vi "LIN To 2SCU.vi"() -> ()   [LabVIEW 2018]
panel:
  in  "NAD":u8[](array[numeric])=[13, 120] format="%.0x"
  in  "关闭卷帘":bool
  in  "展开卷帘":bool
  in  "关闭天窗":bool
  in  "打开天窗":bool
  in  "Send":bool
  out "Tx Rx Data":string
  out "Response Good?":bool
  in  "Exit":bool
  in  "interface":refnum<k21>="LIN2"
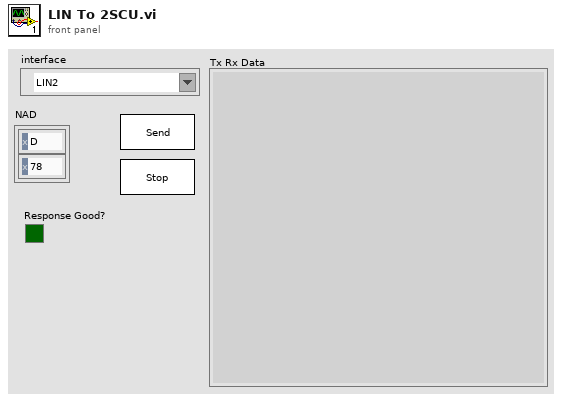
[diagram p1: front panel]
types:
  T1 = typedef "LIN Device.ctl" = cluster{"Master Frame(3C)":refnum<k21>, "Slave Frame(3D)":refnum<k21>, "Request Schedule":refnum<k21>, "Response Schedule":refnum<k21>, "Frame Write SCU":refnum<k21>, "Frame Read SCU":refnum<k21>, "LIN Name":refnum<k21>}
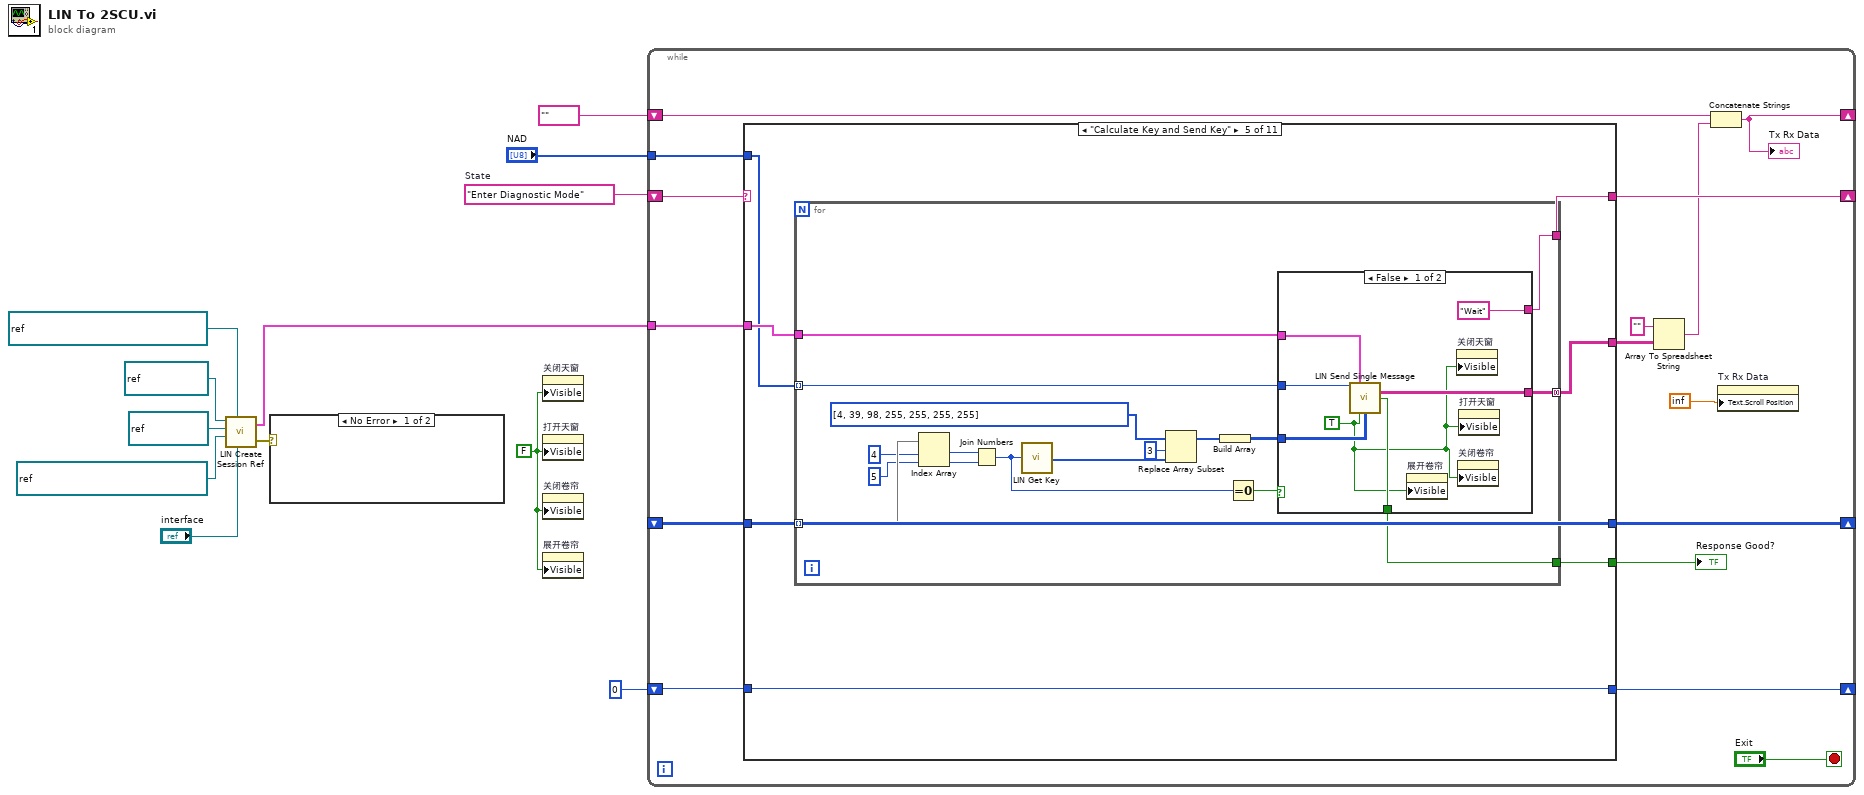
[diagram p0: block diagram]
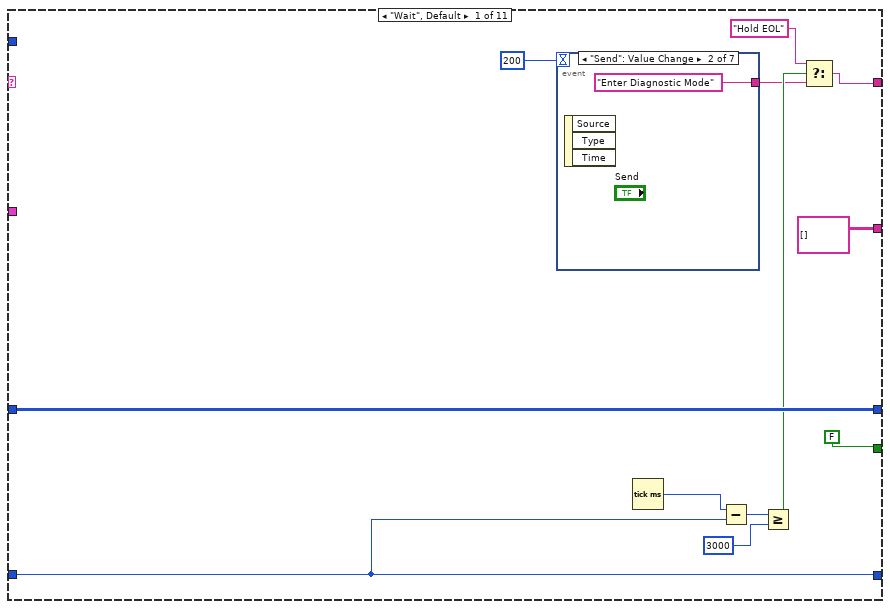
[diagram p2: hidden frame]
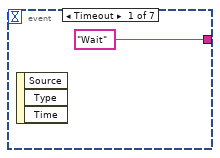
[diagram p3: hidden frame]
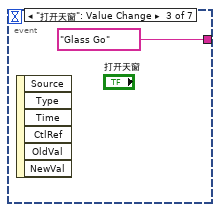
[diagram p4: hidden frame]
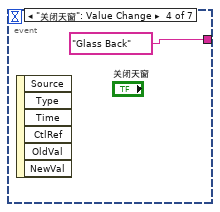
[diagram p5: hidden frame]
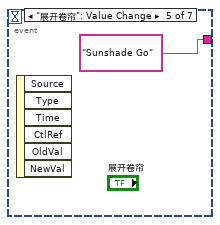
[diagram p6: hidden frame]
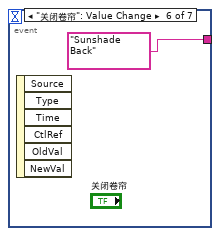
[diagram p7: hidden frame]
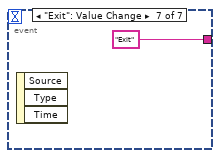
[diagram p8: hidden frame]
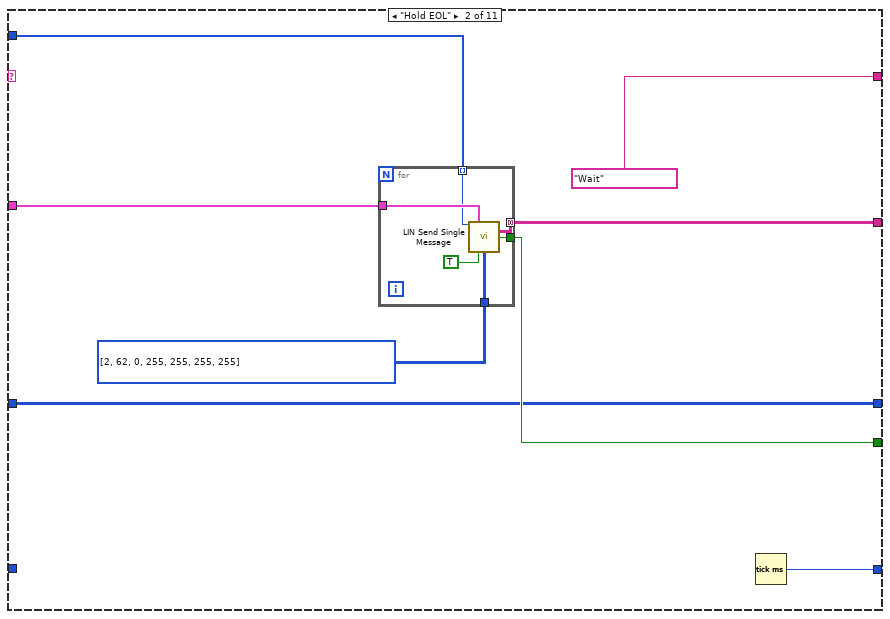
[diagram p9: hidden frame]
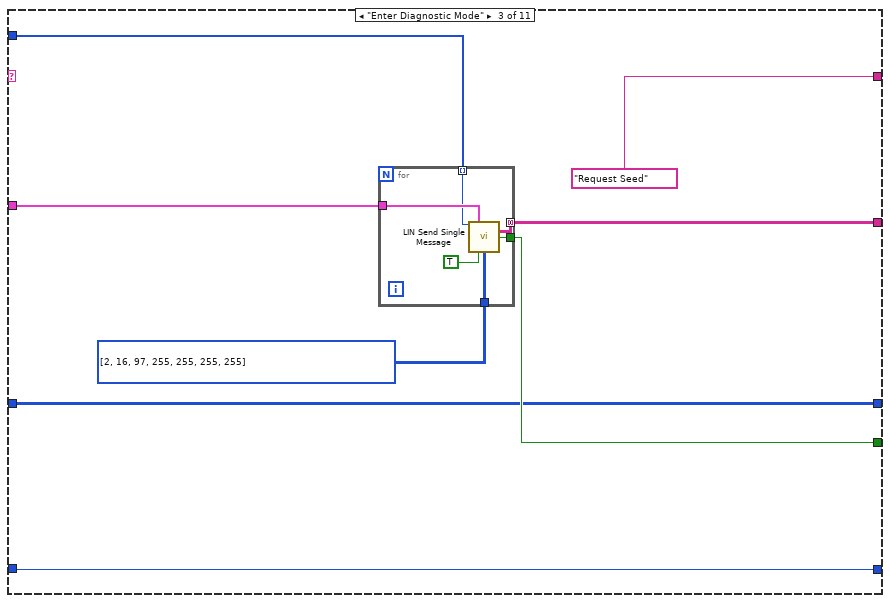
[diagram p10: hidden frame]
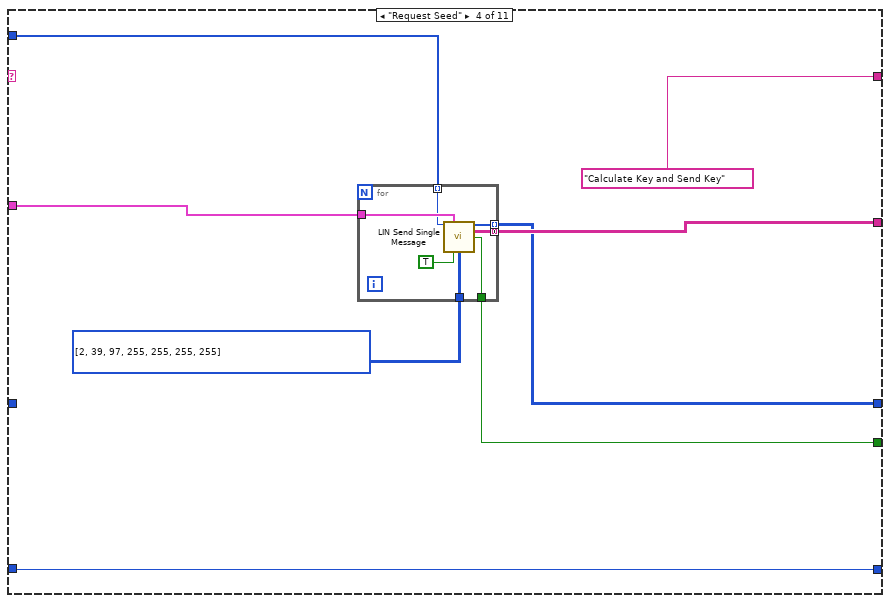
[diagram p11: hidden frame]
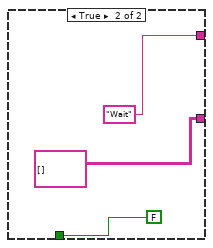
[diagram p12: hidden frame]
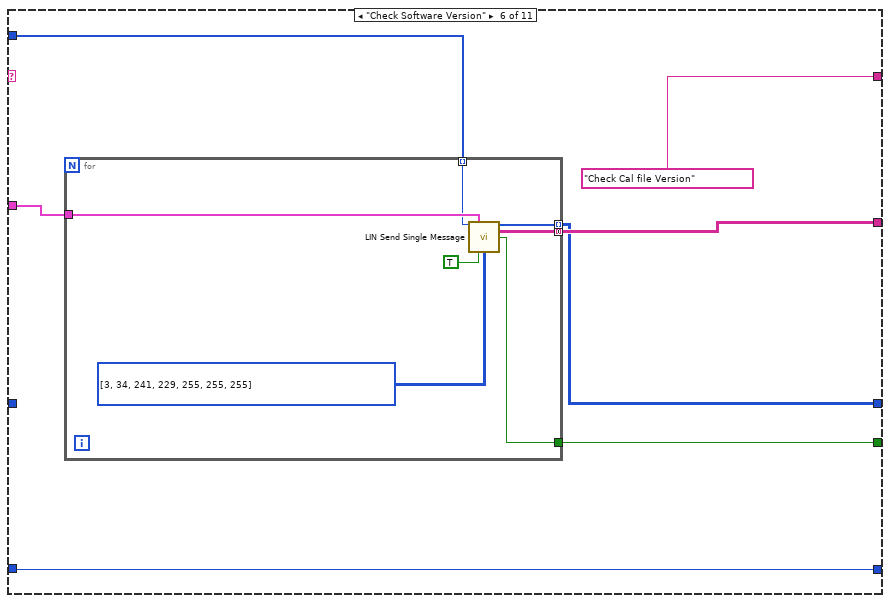
[diagram p13: hidden frame]
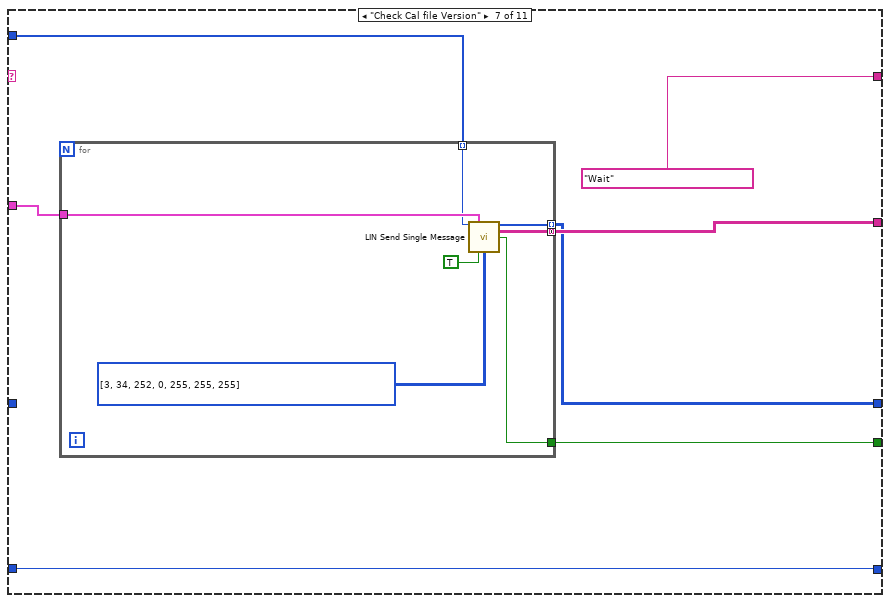
[diagram p14: hidden frame]
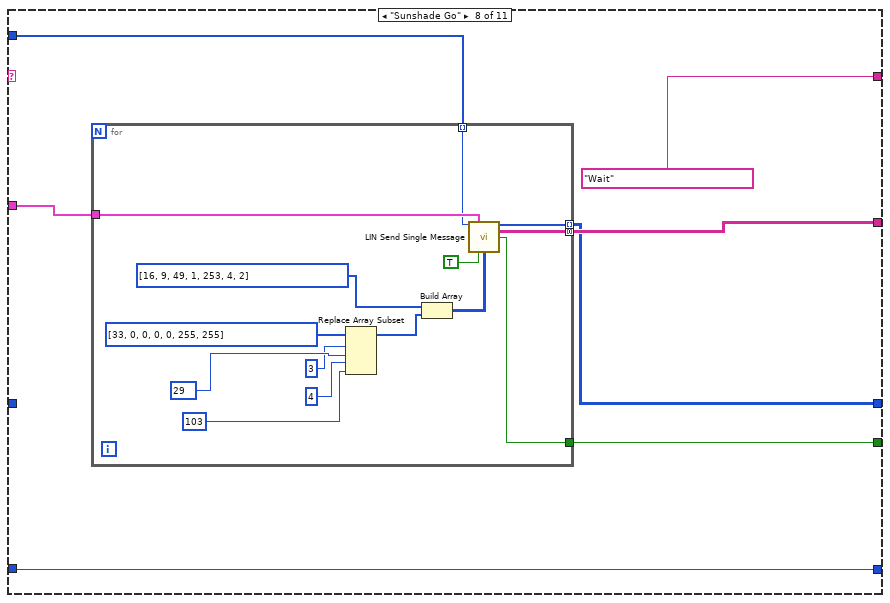
[diagram p15: hidden frame]
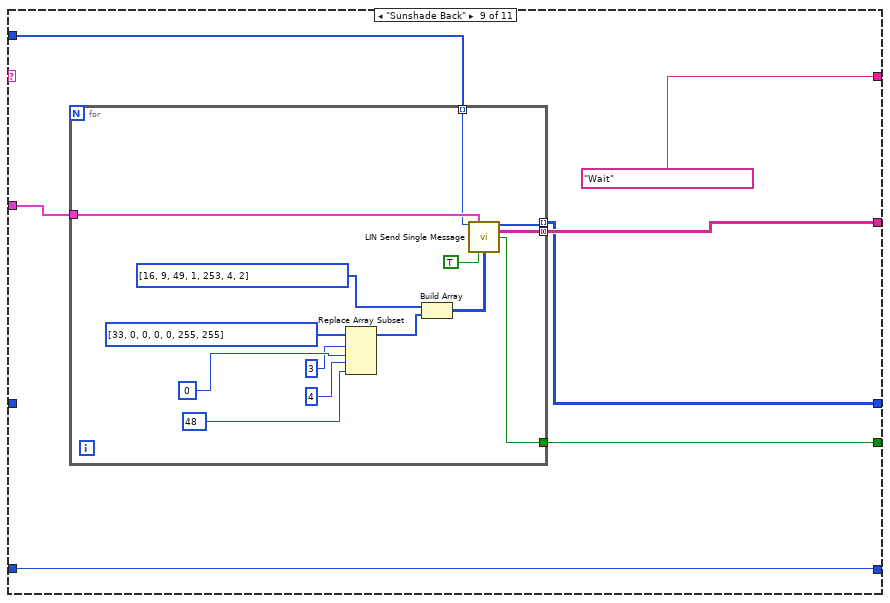
[diagram p16: hidden frame]
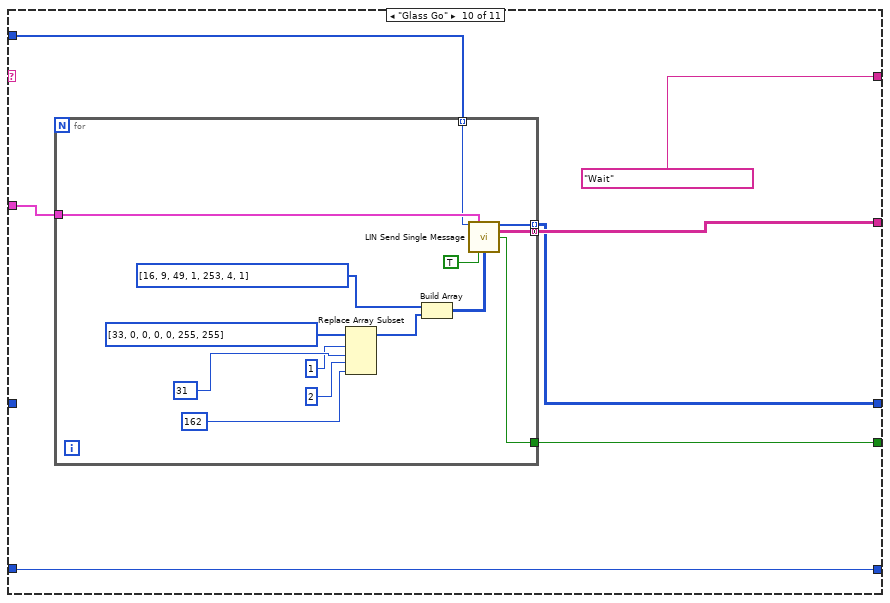
[diagram p17: hidden frame]
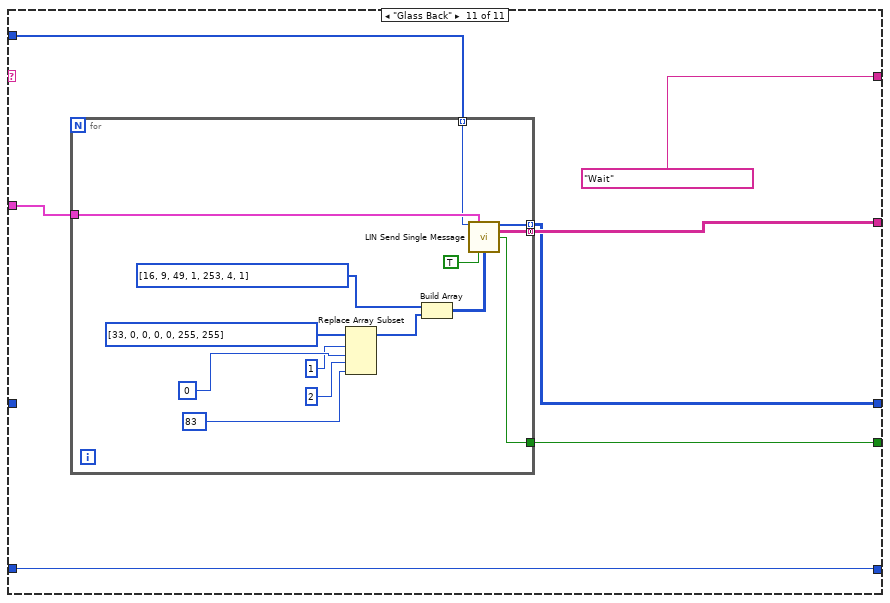
[diagram p18: hidden frame]
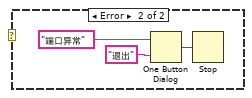
[diagram p19: hidden frame]
diagram:
  w3 = FALSE
  w6 = "Enter Diagnostic Mode"  # State
  n1 = call "LIN Create Session Ref.vi"("interface"="interface", "Response Schedule"=refnum<k21> "CEMLIN3DiagResponseSchedule\nCS110501", "Request Schedule"=refnum<k21> "CEMLIN3DiagRequestSchedule\nCS110501", "Slave Frame(3D)"=refnum<k21> "SlaveResp\nCS110501", "Master Frame(3C)"=refnum<k21> "MasterReq\nCS110501") -> ("错误输出"=w7:errorcluster, "LIN Device"=w4:T1)  [unwired: 1 in]
  n2 = case shown="No Error" w7 {
    frame No Error {
    }
    frame Error {
      n3 = One Button Dialog(message="端口异常" ("消息"), button name ("OK")="退出" ("按钮名称（“确定”）")) -> (true=w13:bool)
      n4 = Stop(stop? (T)=w13) -> ()
    }
  }
  n5 = property on="关闭天窗" class="Bool"("Visible"=w3) -> ()  [unwired: 2 in, 2 out]
  n6 = property on="打开天窗" class="Bool"("Visible"=w3) -> ()  [unwired: 2 in, 2 out]
  n7 = property on="关闭卷帘" class="Bool"("Visible"=w3) -> ()  [unwired: 2 in, 2 out]
  n8 = property on="展开卷帘" class="Bool"("Visible"=w3) -> ()  [unwired: 2 in, 2 out]
  n9 = while {
    shift-right: [w29] -> _
    shift-left: w6 -> [w31]
    shift-right: [w24] -> _
    shift-left: "" -> [w25]
    shift-right: [w22] -> _
    shift-left: _ -> [w30]
    tunnel: w4 -> [w23]
    tunnel: "NAD" -> [w18]
    shift-right: [w16] -> _
    shift-left: u32 0 ("millisecond timer value") -> [w17]
    stop <- "Exit" stop-if-true
    n10 = case shown="\"Calculate Key and Send Key\"" w31 {
      tunnel: w30 -> [w40 w53 w67 _ w100 _ _ _ _ _ _]
      tunnel: [w34 "Wait" "Request Seed" "Calculate Key and Send Key" w97 "Check Cal file Version" "Wait" "Wait" "Wait" "Wait" "Wait"] -> w29
      tunnel: [string[][] [] ("TxRx Data") w56 w70 w84 w98 w133 w147 w161 w182 w203 w224] -> w28
      tunnel: w23 -> [_ w57 w71 w85 w99 w134 w148 w162 w183 w204 w225]
      tunnel: [w40 w53 w67 w82 w100 w131 w145 w159 w180 w201 w222] -> w22
      tunnel: [FALSE w54 w68 w81 w96 w130 w144 w158 w179 w200 w221] -> w21
      tunnel: w18 -> [_ w52 w66 w80 w95 w129 w143 w157 w178 w199 w220]
      tunnel: w17 -> [w32 _ w65 w79 w94 w128 w142 w156 w177 w198 w219]
      tunnel: [w32 w51 w65 w79 w94 w128 w142 w156 w177 w198 w219] -> w16
      frame "Wait", Default {
        n11 = event shown="[1] \"Send\": Value Change" {
          selector: _ -> [_ _ _ _ _ _ _]
          dyn-events: _ -> [_ _ _ _ _ _ _]
          timeout: 200 -> [_ _ _ _ _ _ _]
          tunnel: ["Wait" "Enter Diagnostic Mode" "Glass Go" ("State") "Glass Back" ("State") "Sunshade Go" ("State") "Sunshade Back" ("State") "Exit" ("format string")] -> w35
          event Timeout {
            n12 = event-data() -> ()  [unwired: 1 in, 3 out]
          }
          event "Send": Value Change {
            n13 = event-data() -> ()  [unwired: 1 in, 3 out]
          }
          event "打开天窗": Value Change {
            n14 = event-data() -> ()  [unwired: 1 in, 6 out]
          }
          event "关闭天窗": Value Change {
            n15 = event-data() -> ()  [unwired: 1 in, 6 out]
          }
          event "展开卷帘": Value Change {
            n16 = event-data() -> ()  [unwired: 1 in, 6 out]
          }
          event "关闭卷帘": Value Change {
            n17 = event-data() -> ()  [unwired: 1 in, 6 out]
          }
          event "Exit": Value Change {
            n18 = event-data() -> ()  [unwired: 1 in, 3 out]
          }
        }
        n19 = Tick Count (ms)() -> (millisecond timer value=w39:u32)
        n20 = Subtract(x=w39, y=w32) -> (x-y=w38:u32)
        n21 = Greater Or Equal?(x=w38, y=u32 3000) -> (x >= y?=w36:bool)
        n22 = Select(t="Hold EOL", s=w36, f=w35) -> (s? t:f=w34:string)
      }
      frame "Hold EOL" {
        n23 = for {
          tunnel: u8[][] [[2, 62, 0, 255, 255, 255, 255]] -> [w64]
          tunnel: w57 -> [w63]
          tunnel: [w62] -> w56 mode=concatenating
          tunnel: [w61] -> w54
          tunnel: w52 -> [w59] mode=indexing
          n24 = call "LIN Send Single Message.vi"("NAD"=w59, "LIN Device"=w63, "Need REQ"=TRUE, "Tx Msg"=w64) -> ("TxRx Data"=w62:string[][], "Response Good?"=w61:bool)  [unwired: 6 in, 4 out]
        }
        n25 = Tick Count (ms)() -> (millisecond timer value=w51:u32)
      }
      frame "Enter Diagnostic Mode" {
        n26 = for {
          tunnel: u8[][] [[2, 16, 97, 255, 255, 255, 255]] -> [w78]
          tunnel: w71 -> [w77]
          tunnel: [w76] -> w70 mode=concatenating
          tunnel: [w75] -> w68
          tunnel: w66 -> [w73] mode=indexing
          n27 = call "LIN Send Single Message.vi"("NAD"=w73, "LIN Device"=w77, "Need REQ"=TRUE, "Tx Msg"=w78) -> ("TxRx Data"=w76:string[][], "Response Good?"=w75:bool)  [unwired: 6 in, 4 out]
        }
      }
      frame "Request Seed" {
        n28 = for {
          tunnel: u8[][] [[2, 39, 97, 255, 255, 255, 255]] -> [w93]
          tunnel: w85 -> [w92]
          tunnel: [w91] -> w84 mode=concatenating
          tunnel: [w90] -> w82 mode=indexing
          tunnel: [w89] -> w81
          tunnel: w80 -> [w87] mode=indexing
          n29 = call "LIN Send Single Message.vi"("NAD"=w87, "LIN Device"=w92, "Need REQ"=TRUE, "Tx Msg"=w93) -> ("Rx Msg"=w90:u8[], "TxRx Data"=w91:string[][], "Response Good?"=w89:bool)  [unwired: 6 in, 3 out]
        }
      }
      frame "Calculate Key and Send Key" {
        n30 = for {
          tunnel: w100 -> [w117] mode=indexing
          tunnel: w99 -> [w105]
          tunnel: [w104] -> w98 mode=concatenating
          tunnel: [w103] -> w97
          tunnel: [w102] -> w96
          tunnel: w95 -> [w101] mode=indexing
          n31 = Index Array(array=w117, index #1=4 ("索引"), index #2=5 ("索引")) -> (element #1=w114:u8, element #2=w113:u8)
          n32 = Join Numbers(hi=w114, lo=w113) -> ((hi.lo)=w107:u16)
          n33 = call "LIN Get Key.vi"("x"=w107) -> ("KEY"=w111:u8[])
          n34 = Replace Array Subset(array=u8[] [4, 39, 98, 255, 255, 255, 255], new element=w111, index=3 ("索引")) -> (w109:u8[])
          n35 = Build Array(w109) -> (w106:u8[][])
          n36 = Equal To 0?(x=w107) -> (x = 0?=w108:bool)
          n37 = case shown="False" w108 {
            tunnel: w106 -> [w124 _]
            tunnel: w105 -> [w123 _]
            tunnel: [w122 string[][] [] ("TxRx Data")] -> w104
            tunnel: ["Wait" ("format string") "Wait" ("format string")] -> w103
            tunnel: [w120 FALSE ("Response Good?")] -> w102
            tunnel: w101 -> [w118 _]
            frame False {
              w119 = TRUE ("Need REQ")
              n38 = call "LIN Send Single Message.vi"("NAD"=w118, "LIN Device"=w123, "Need REQ"=w119, "Tx Msg"=w124) -> ("TxRx Data"=w122:string[][], "Response Good?"=w120:bool)  [unwired: 6 in, 4 out]
              n39 = property on="展开卷帘" class="Bool"("Visible"=w119) -> ()  [unwired: 2 in, 2 out]
              n40 = property on="关闭天窗" class="Bool"("Visible"=w119) -> ()  [unwired: 2 in, 2 out]
              n41 = property on="关闭卷帘" class="Bool"("Visible"=w119) -> ()  [unwired: 2 in, 2 out]
              n42 = property on="打开天窗" class="Bool"("Visible"=w119) -> ()  [unwired: 2 in, 2 out]
            }
            frame True {
            }
          }
        }
      }
      frame "Check Software Version" {
        n43 = for {
          tunnel: w134 -> [w140]
          tunnel: [w139] -> w133 mode=concatenating
          tunnel: [w138] -> w131 mode=indexing
          tunnel: [w137] -> w130
          tunnel: w129 -> [w135] mode=indexing
          n44 = call "LIN Send Single Message.vi"("NAD"=w135, "LIN Device"=w140, "Need REQ"=TRUE, "Tx Msg"=u8[][] [[3, 34, 241, 229, 255, 255, 255]]) -> ("Rx Msg"=w138:u8[], "TxRx Data"=w139:string[][], "Response Good?"=w137:bool)  [unwired: 6 in, 3 out]
        }
      }
      frame "Check Cal file Version" {
        n45 = for {
          tunnel: w148 -> [w154]
          tunnel: [w153] -> w147 mode=concatenating
          tunnel: [w152] -> w145 mode=indexing
          tunnel: [w151] -> w144
          tunnel: w143 -> [w149] mode=indexing
          n46 = call "LIN Send Single Message.vi"("NAD"=w149, "LIN Device"=w154, "Need REQ"=TRUE, "Tx Msg"=u8[][] [[3, 34, 252, 0, 255, 255, 255]]) -> ("Rx Msg"=w152:u8[], "TxRx Data"=w153:string[][], "Response Good?"=w151:bool)  [unwired: 6 in, 3 out]
        }
      }
      frame "Sunshade Go" {
        n47 = for {
          tunnel: w162 -> [w176]
          tunnel: [w175] -> w161 mode=concatenating
          tunnel: [w174] -> w159 mode=indexing
          tunnel: [w173] -> w158
          tunnel: w157 -> [w163] mode=indexing
          n48 = Replace Array Subset(array=u8[] [33, 0, 0, 0, 0, 255, 255], new element #1=29 ("Go to Position"), index #1=3 ("index"), new element #2=103 ("Go to Position"), index #2=4 ("index")) -> (w165:u8[])
          n49 = Build Array(u8[] [16, 9, 49, 1, 253, 4, 2], w165) -> (w164:u8[][])
          n50 = call "LIN Send Single Message.vi"("NAD"=w163, "LIN Device"=w176, "Need REQ"=TRUE, "Tx Msg"=w164) -> ("Rx Msg"=w174:u8[], "TxRx Data"=w175:string[][], "Response Good?"=w173:bool)  [unwired: 6 in, 3 out]
        }
      }
      frame "Sunshade Back" {
        n51 = for {
          tunnel: w183 -> [w197]
          tunnel: [w196] -> w182 mode=concatenating
          tunnel: [w195] -> w180 mode=indexing
          tunnel: [w194] -> w179
          tunnel: w178 -> [w184] mode=indexing
          n52 = Replace Array Subset(array=u8[] [33, 0, 0, 0, 0, 255, 255], new element #1=0 ("Go to Position"), index #1=3 ("index"), new element #2=48 ("Go to Position"), index #2=4 ("index")) -> (w186:u8[])
          n53 = Build Array(u8[] [16, 9, 49, 1, 253, 4, 2], w186) -> (w185:u8[][])
          n54 = call "LIN Send Single Message.vi"("NAD"=w184, "LIN Device"=w197, "Need REQ"=TRUE, "Tx Msg"=w185) -> ("Rx Msg"=w195:u8[], "TxRx Data"=w196:string[][], "Response Good?"=w194:bool)  [unwired: 6 in, 3 out]
        }
      }
      frame "Glass Go" {
        n55 = for {
          tunnel: w204 -> [w218]
          tunnel: [w217] -> w203 mode=concatenating
          tunnel: [w216] -> w201 mode=indexing
          tunnel: [w215] -> w200
          tunnel: w199 -> [w205] mode=indexing
          n56 = Replace Array Subset(array=u8[] [33, 0, 0, 0, 0, 255, 255], new element #1=31 ("Go to Position"), index #1=1 ("index"), new element #2=162 ("Go to Position"), index #2=2 ("index")) -> (w207:u8[])
          n57 = Build Array(u8[] [16, 9, 49, 1, 253, 4, 1], w207) -> (w206:u8[][])
          n58 = call "LIN Send Single Message.vi"("NAD"=w205, "LIN Device"=w218, "Need REQ"=TRUE, "Tx Msg"=w206) -> ("Rx Msg"=w216:u8[], "TxRx Data"=w217:string[][], "Response Good?"=w215:bool)  [unwired: 6 in, 3 out]
        }
      }
      frame "Glass Back" {
        n59 = for {
          tunnel: w225 -> [w239]
          tunnel: [w238] -> w224 mode=concatenating
          tunnel: [w237] -> w222 mode=indexing
          tunnel: [w236] -> w221
          tunnel: w220 -> [w226] mode=indexing
          n60 = Replace Array Subset(array=u8[] [33, 0, 0, 0, 0, 255, 255], new element #1=0 ("Go to Position"), index #1=1 ("index"), new element #2=83 ("Go to Position"), index #2=2 ("index")) -> (w228:u8[])
          n61 = Build Array(u8[] [16, 9, 49, 1, 253, 4, 1], w228) -> (w227:u8[][])
          n62 = call "LIN Send Single Message.vi"("NAD"=w226, "LIN Device"=w239, "Need REQ"=TRUE, "Tx Msg"=w227) -> ("Rx Msg"=w237:u8[], "TxRx Data"=w238:string[][], "Response Good?"=w236:bool)  [unwired: 6 in, 3 out]
        }
      }
    }
    "Response Good?" <- w21
    n63 = Array To Spreadsheet String(array=w28, 3:"" ("格式字符串")) -> (spreadsheet string=w26:string)  [unwired: 1 in]
    n64 = Concatenate Strings(w25, w26) -> (w24:string)
    "Tx Rx Data" <- w24
    n65 = property on="Tx Rx Data" class="Str"("Text.Scroll Position"=inf) -> ()  [unwired: 2 in, 2 out]
  }
